vi "Run_3_of_6_Tests.vi"() -> ()   [LabVIEW 2019]
uses:
  <vilib>/Rock Robotics/WPI/ThirdParty/JAS_Junk/TrajLib/Trajectory_Library.lvlib
panel:
  out "Rectangular Region\nConstraint":bool
  out "String":string
  out "Profiled PID Input/Output":bool
  out "State Space Util":bool
  out "Runge Kutta Time Varying":bool
  out "Swerve Drive Kinematics":bool
  out "Swerve Drive Odometry":bool
  out "All Tests Finished":bool
  out "Trajectory Concatenate":bool
  out "Timer":bool
  out "Single Jointed Arm Sim":bool
  out "Simple Motor Feedforward":bool
  out "Swerve Drive Pose Est":bool
  out "Swerve Module State":bool
  out "Slew Rate Limiter":bool
  out "Quintic Spline":bool
  out "Ramsete":bool
  out "Profiled PID":bool
  out "Rotation2d":bool
  out "Pose2d":bool
  out "PID tolerance":bool
  # "FORMAL TRAJECTORY / CONTROL LIBRARY TEST PROCEDURE"
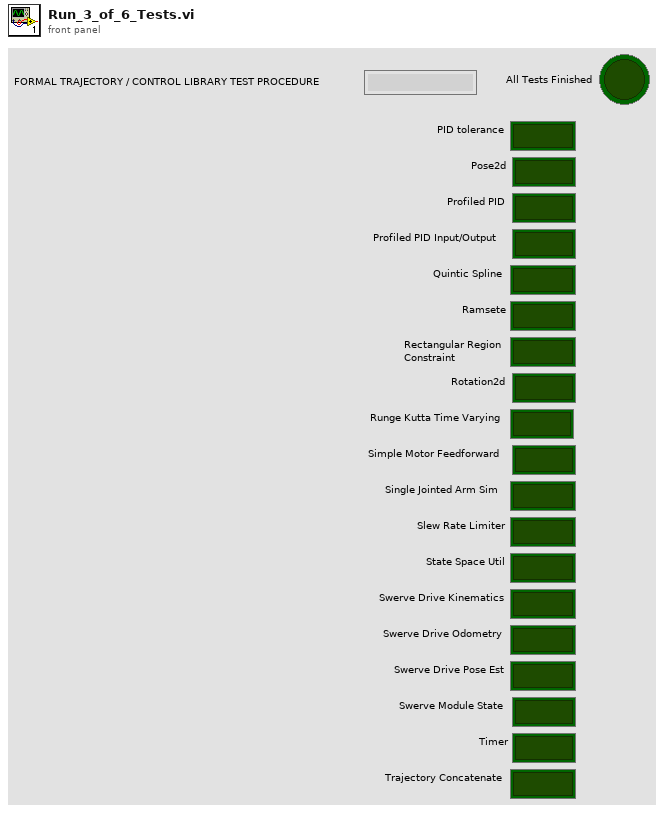
[diagram p1: front panel]
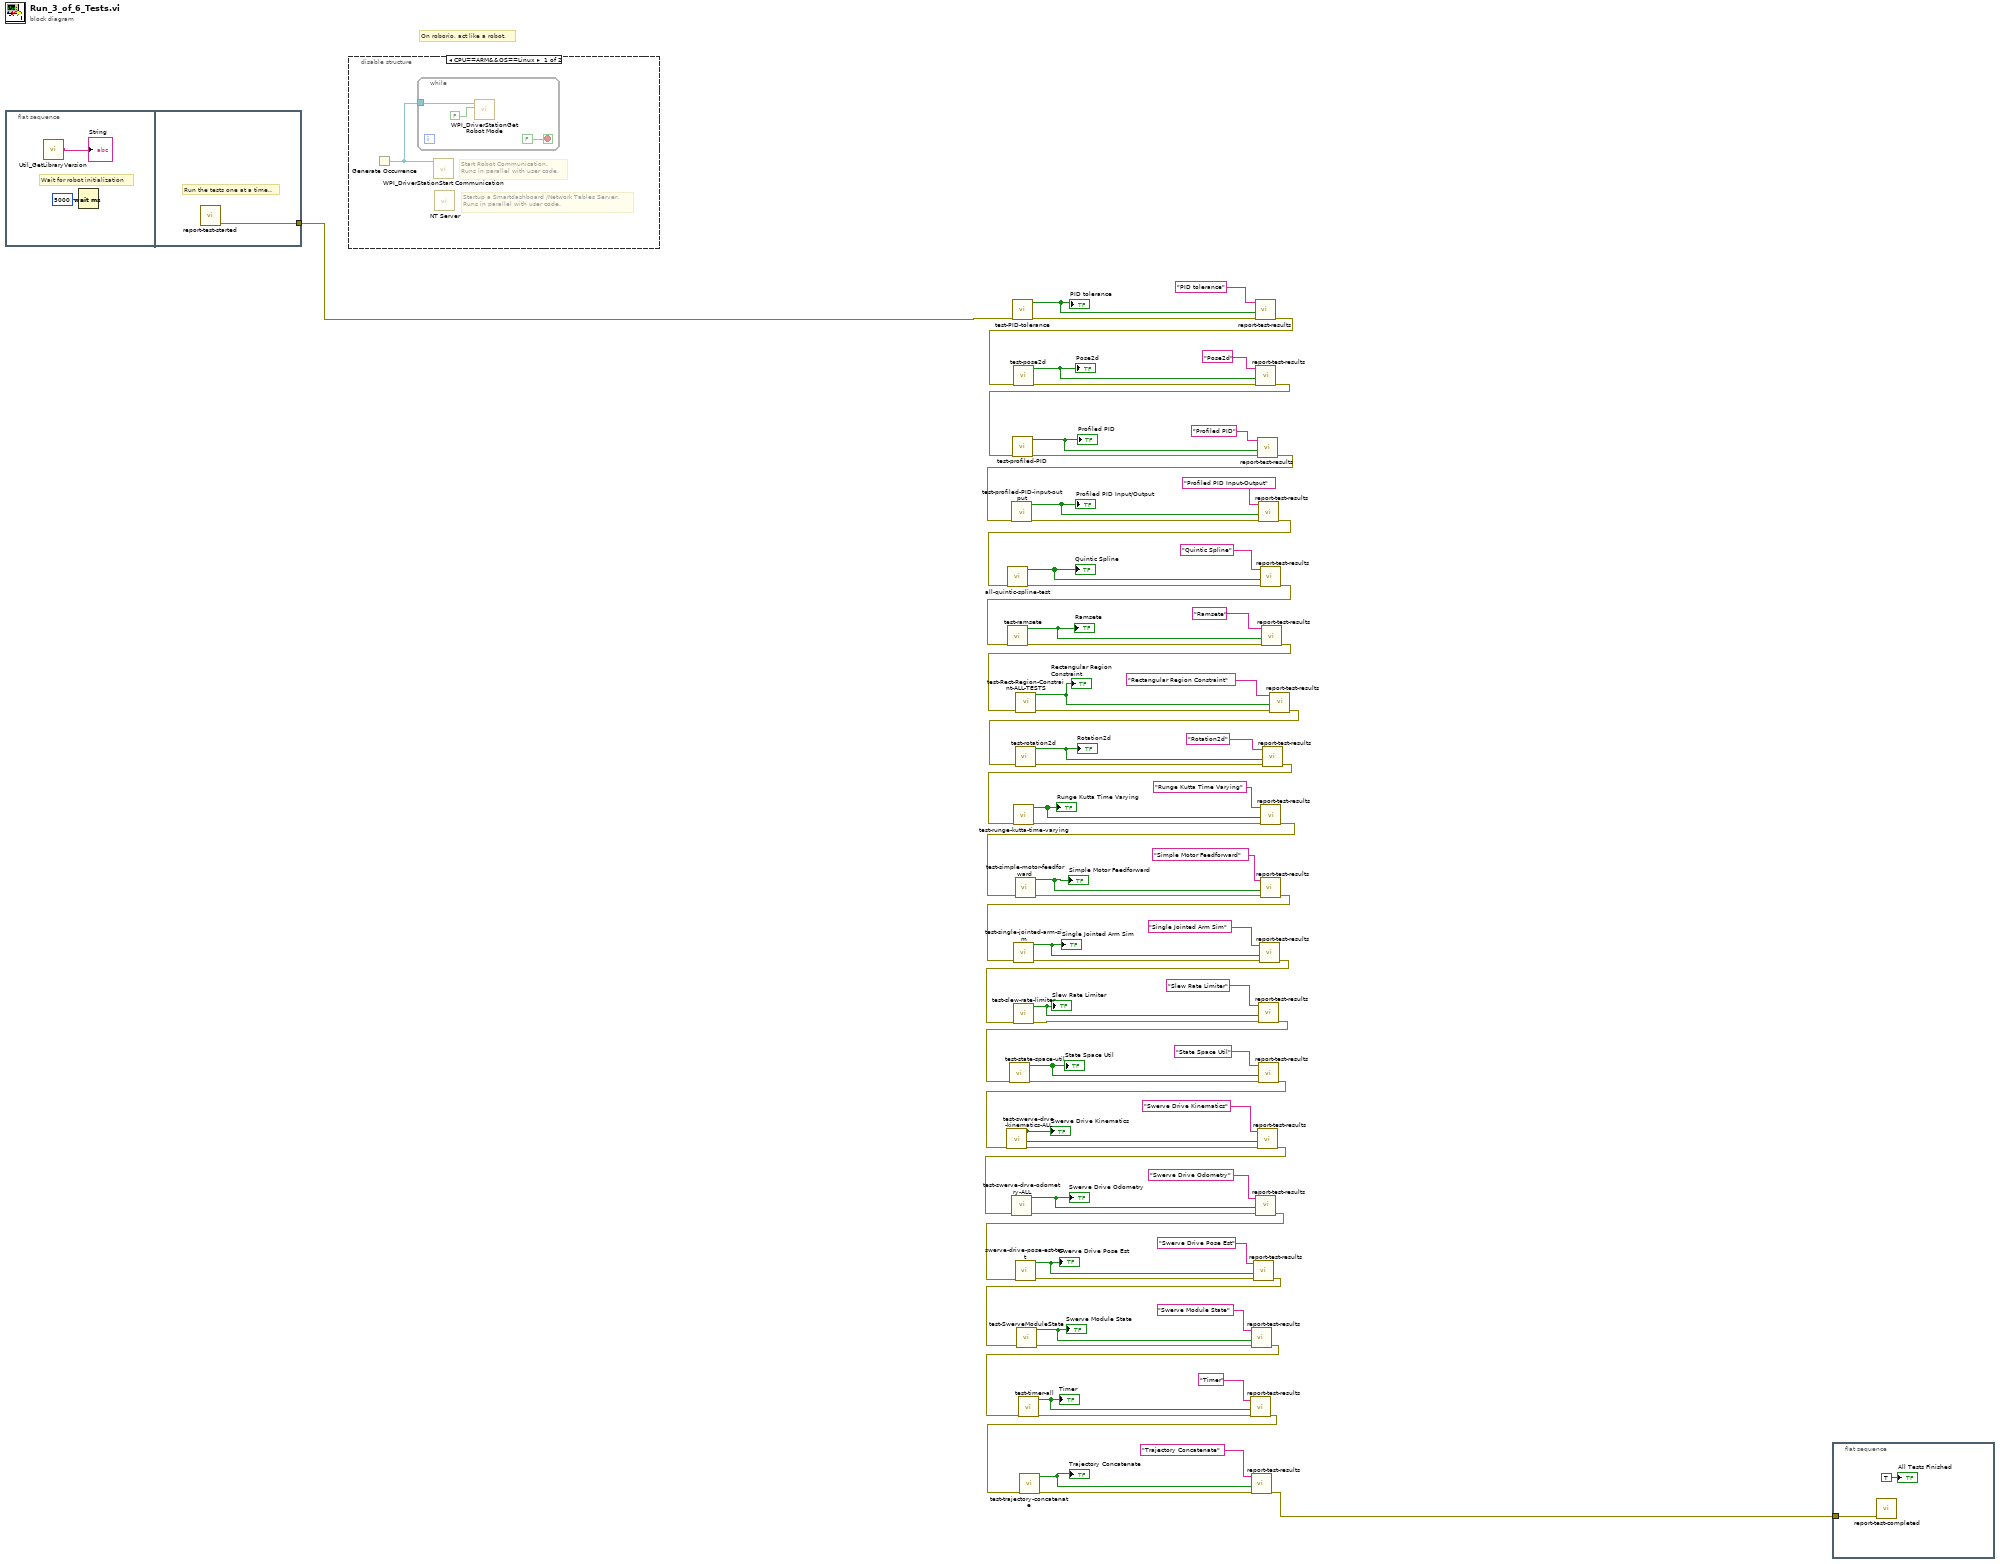
[diagram p0: block diagram]
diagram:
  # "On roborio, act like a robot."
  n1 = flat-sequence {
    tunnel: [w80] -> w6
    frame #0 {
      # "Wait for robot initialization"
      n2 = call <vilib>:"Util_GetLibraryVersion.vi"() -> ("TrajLibVersion"=→"String":string)  [unwired: 11 in]
      n3 = Wait (ms)(milliseconds to wait=u32 5000) -> ()  [unwired: 1 out]
    }
    frame #1 {
      # "Run the tests one at a time.."
      n4 = call "report-test-started.vi"() -> ("error out"=w80:errorcluster)  [unwired: 11 in]
    }
  }
  n5 = disable-structure shown="CPU==ARM&&OS==Linux" {
    frame condition #0 {
      # "Startup a Smartdashboard /Network Tables Server.\nRuns in parallel with user code."
      # "Start Robot Communication.\nRuns in parallel with user code."
      n6 = Generate Occurrence() -> (w81:refnum<k4>)
      n7 = while {
        tunnel: w81 -> [w84]
        stop <- FALSE stop-if-true
        n8 = call <vilib>:"WPI_DriverStationGet Robot Mode.vi"("Finish"=FALSE, "DS Occurrence"=w84) -> ()  [unwired: 10 out]
      }
      n9 = call <vilib>:"WPI_DriverStationStart Communication.vi"("occurrence"=w81) -> ()  [unwired: 2 in, 9 out]
      n10 = call <vilib>:"NT Server.vi"() -> ()  [unwired: 12 in]
    }
    frame condition #1 (active) {
    }
  }
  n11 = call "test-PID-tolerance.vi"("error in (no error)"=w6) -> ("error out"=w41:errorcluster, "All Tests Passed"=w74:bool)  [unwired: 9 in]
  "PID tolerance" <- w74
  n12 = call "report-test-results.vi"("error in (no error)"=w41, "TestPassed"=w74, "Test Name"="PID tolerance") -> ("error out"=w23:errorcluster)  [unwired: 8 in]
  n13 = call "test-pose2d.vi"("error in (no error)"=w23) -> ("error out"=w40:errorcluster, "All PASSED"=w75:bool)  [unwired: 9 in]
  "Pose2d" <- w75
  n14 = call "report-test-results.vi"("error in (no error)"=w40, "TestPassed"=w75, "Test Name"="Pose2d") -> ("error out"=w38:errorcluster)  [unwired: 8 in]
  n15 = call "test-profiled-PID.vi"("error in (no error)"=w38) -> ("error out"=w39:errorcluster, "Test Passed 0"=w62:bool)  [unwired: 9 in]
  "Profiled PID" <- w62
  n16 = call "report-test-results.vi"("error in (no error)"=w39, "TestPassed"=w62, "Test Name"="Profiled PID") -> ("error out"=w22:errorcluster)  [unwired: 8 in]
  n17 = call "test-profiled-PID-input-output.vi"("error in (no error)"=w22) -> ("error out"=w37:errorcluster, "All Tests Passed"=w61:bool)  [unwired: 9 in]
  "Profiled PID Input/Output" <- w61
  n18 = call "report-test-results.vi"("error in (no error)"=w37, "TestPassed"=w61, "Test Name"="Profiled PID Input-Output") -> ("error out"=w21:errorcluster)  [unwired: 8 in]
  n19 = call "all-quintic-spline-test.vi"("error in (no error)"=w21) -> ("error out"=w36:errorcluster, "ALL TESTS PASSED"=w60:bool)  [unwired: 9 in]
  "Quintic Spline" <- w60
  n20 = call "report-test-results.vi"("error in (no error)"=w36, "TestPassed"=w60, "Test Name"="Quintic Spline") -> ("error out"=w20:errorcluster)  [unwired: 8 in]
  n21 = call "test-ramsete.vi"("error in (no error)"=w20) -> ("error out"=w24:errorcluster, "AtReference End"=w59:bool)  [unwired: 9 in]
  "Ramsete" <- w59
  n22 = call "report-test-results.vi"("error in (no error)"=w24, "TestPassed"=w59, "Test Name"="Ramsete") -> ("error out"=w2:errorcluster)  [unwired: 8 in]
  n23 = call "test-Rect-Region-Constraint-ALL-TESTS.vi"("error in (no error)"=w2) -> ("error out"=w4:errorcluster, "All Passed"=w3:bool)  [unwired: 9 in]
  "Rectangular Region\nConstraint" <- w3
  n24 = call "report-test-results.vi"("error in (no error)"=w4, "TestPassed"=w3, "Test Name"="Rectangular Region Constraint") -> ("error out"=w1:errorcluster)  [unwired: 8 in]
  n25 = call "test-rotation2d.vi"("error in (no error)"=w1) -> ("error out"=w25:errorcluster, "ALL TESTS PASSED"=w58:bool)  [unwired: 9 in]
  "Rotation2d" <- w58
  n26 = call "report-test-results.vi"("error in (no error)"=w25, "TestPassed"=w58, "Test Name"="Rotation2d") -> ("error out"=w19:errorcluster)  [unwired: 8 in]
  n27 = call "test-runge-kutta-time-varying.vi"("error in (no error)"=w19) -> ("error out"=w26:errorcluster, "Test Passed"=w57:bool)  [unwired: 9 in]
  "Runge Kutta Time Varying" <- w57
  n28 = call "report-test-results.vi"("error in (no error)"=w26, "TestPassed"=w57, "Test Name"="Runge Kutta Time Varying") -> ("error out"=w18:errorcluster)  [unwired: 8 in]
  n29 = call "test-simple-motor-feedforward.vi"("error in (no error)"=w18) -> ("error out"=w27:errorcluster, "All Tests Passed"=w56:bool)  [unwired: 9 in]
  "Simple Motor Feedforward" <- w56
  n30 = call "report-test-results.vi"("error in (no error)"=w27, "TestPassed"=w56, "Test Name"="Simple Motor Feedforward") -> ("error out"=w17:errorcluster)  [unwired: 8 in]
  n31 = call "test-single-jointed-arm-sim.vi"("error in (no error)"=w17) -> ("error out"=w28:errorcluster, "Test Passed"=w55:bool)  [unwired: 9 in]
  "Single Jointed Arm Sim" <- w55
  n32 = call "report-test-results.vi"("error in (no error)"=w28, "TestPassed"=w55, "Test Name"="Single Jointed Arm Sim") -> ("error out"=w16:errorcluster)  [unwired: 8 in]
  n33 = call "test-slew-rate-limiter.vi"("error in (no error)"=w16) -> ("error out"=w29:errorcluster, "All Tests Passed"=w54:bool)  [unwired: 9 in]
  "Slew Rate Limiter" <- w54
  n34 = call "report-test-results.vi"("error in (no error)"=w29, "TestPassed"=w54, "Test Name"="Slew Rate Limiter") -> ("error out"=w15:errorcluster)  [unwired: 8 in]
  n35 = call "test-state-space-util.vi"("error in (no error)"=w15) -> ("error out"=w30:errorcluster, "All Tests Passed"=w53:bool)  [unwired: 9 in]
  "State Space Util" <- w53
  n36 = call "report-test-results.vi"("error in (no error)"=w30, "TestPassed"=w53, "Test Name"="State Space Util") -> ("error out"=w14:errorcluster)  [unwired: 8 in]
  n37 = call "test-swerve-drve-kinematics-ALL.vi"("error in (no error)"=w14) -> ("error out"=w31:errorcluster, "ALL TEsts Passed"=w52:bool)  [unwired: 9 in]
  "Swerve Drive Kinematics" <- w52
  n38 = call "report-test-results.vi"("error in (no error)"=w31, "TestPassed"=w52, "Test Name"="Swerve Drive Kinematics") -> ("error out"=w13:errorcluster)  [unwired: 8 in]
  n39 = call "test-swerve-drve-odometry-ALL.vi"("error in (no error)"=w13) -> ("error out"=w32:errorcluster, "ALL TEsts Passed"=w49:bool)  [unwired: 9 in]
  "Swerve Drive Odometry" <- w49
  n40 = call "report-test-results.vi"("error in (no error)"=w32, "TestPassed"=w49, "Test Name"="Swerve Drive Odometry") -> ("error out"=w12:errorcluster)  [unwired: 8 in]
  n41 = call "swerve-drive-pose-est-test.vi"("error in (no error)"=w12) -> ("error out"=w33:errorcluster, "Test Passed"=w48:bool)  [unwired: 9 in]
  "Swerve Drive Pose Est" <- w48
  n42 = call "report-test-results.vi"("error in (no error)"=w33, "TestPassed"=w48, "Test Name"="Swerve Drive Pose Est") -> ("error out"=w11:errorcluster)  [unwired: 8 in]
  n43 = call "test-SwerveModuleState.vi"("error in (no error)"=w11) -> ("error out"=w34:errorcluster, "ALL TESTS PASSED"=w44:bool)  [unwired: 9 in]
  "Swerve Module State" <- w44
  n44 = call "report-test-results.vi"("error in (no error)"=w34, "TestPassed"=w44, "Test Name"="Swerve Module State") -> ("error out"=w10:errorcluster)  [unwired: 8 in]
  n45 = call "test-timer-all.vi"("error in (no error)"=w10) -> ("error out"=w9:errorcluster, "ALL TESTS PASSED"=w43:bool)  [unwired: 9 in]
  "Timer" <- w43
  n46 = call "report-test-results.vi"("error in (no error)"=w9, "TestPassed"=w43, "Test Name"="Timer") -> ("error out"=w8:errorcluster)  [unwired: 8 in]
  n47 = call "test-trajectory-concatenate.vi"("error in (no error)"=w8) -> ("error out"=w35:errorcluster, "TEsts Passed"=w42:bool)  [unwired: 9 in]
  "Trajectory Concatenate" <- w42
  n48 = call "report-test-results.vi"("error in (no error)"=w35, "TestPassed"=w42, "Test Name"="Trajectory Concatenate") -> ("error out"=w7:errorcluster)  [unwired: 8 in]
  n49 = flat-sequence {
    tunnel: w7 -> [w85]
    frame #0 {
      n50 = call "report-test-completed.vi"("error in (no error)"=w85) -> ()  [unwired: 10 in, 1 out]
      "All Tests Finished" <- TRUE ("All Tests Finished")
    }
  }
